vi "Calc_Number_Chunks.vi"(0 "[IN] U16 Pixel Img":u16[][](array[numeric])) -> (1 "[OUT] Number of chunks":i32, 2 "[OUT] # rows single transfer":i32, 3 "[OUT] # rows last transfer":i32, 4 "[OUT] Not-equal last transfer":bool)   [LabVIEW 2020]
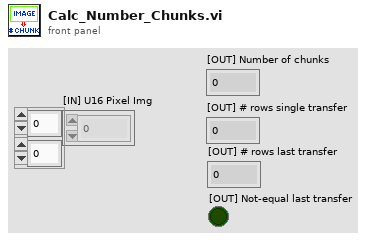
[diagram p1: front panel]
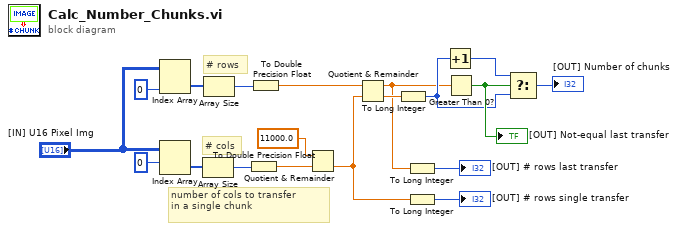
[diagram p0: block diagram]
diagram:
  # "number of cols to transfer \nin a single chunk"
  # "# cols"
  # "# rows"
  n1 = Index Array(array="[IN] U16 Pixel Img", index (col)=0 ("disabled index (col)")) -> (element=w18:u16[])  [unwired: 1 in]
  n2 = Index Array(array="[IN] U16 Pixel Img", index (row)=0 ("disabled index (col)")) -> (element=w15:u16[])  [unwired: 1 in]
  n3 = Array Size(array=w15) -> (size(s)=w13:i32)
  n4 = Array Size(array=w18) -> (size(s)=w14:i32)
  n5 = To Double Precision Float(number=w13) -> (double precision float=w11:dbl)
  n6 = To Double Precision Float(number=w14) -> (double precision float=w10:dbl)
  n7 = Quotient & Remainder(x=11000.0, y=w11) -> (floor(x/y)=w4:dbl)  [unwired: 1 out]
  n8 = Quotient & Remainder(x=w10, y=w4) -> (x-y*floor(x/y)=w2:dbl, floor(x/y)=w8:dbl)
  n9 = To Long Integer(number=w8) -> (32bit integer=w7:i32)
  n10 = To Long Integer(number=w2) -> (32bit integer=→"[OUT] # rows last transfer":i32)
  n11 = To Long Integer(number=w4) -> (32bit integer=→"[OUT] # rows single transfer":i32)
  n12 = Increment(x=w7) -> (x+1=w6:i32)
  n13 = Greater Than 0?(x=w2) -> (x > 0?=w9:bool)
  "[OUT] Not-equal last transfer" <- w9
  n14 = Select(t=w6, s=w9, f=w7) -> (s? t:f=→"[OUT] Number of chunks":i32)
